vi "RH_PPMU_SetVoltage.vi"(8 "error in":errorcluster, 9 "voltage level (V)":dbl, 10 "channel list":string, 11 "PPMU Session In":refnum<k15>) -> (0 "error out":errorcluster, 3 "PPMU Session Out":refnum<k15>)   [LabVIEW 2023, in "ResourceHandling.lvlib"]
doc: "Set Voltage level"
uses:
  ResourceHandling.lvlib
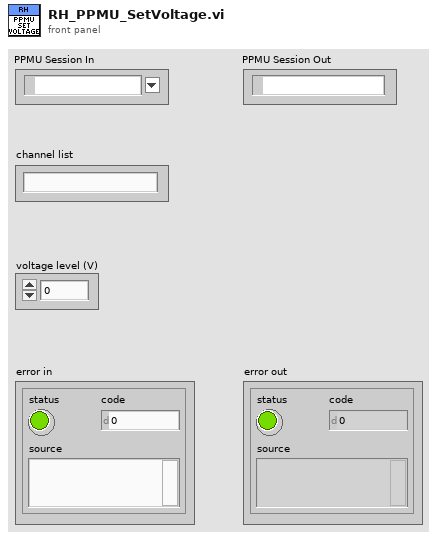
[diagram p1: front panel]
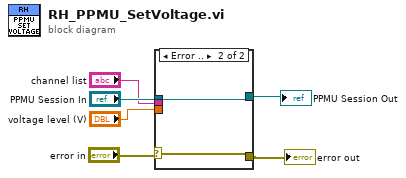
[diagram p0: block diagram]
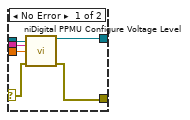
[diagram p2: hidden frame]
diagram:
  n1 = case shown="Error .." "error in" {
    selector: "error in" -> [w9 w13]
    tunnel: "PPMU Session In" -> [w12 w14]
    tunnel: "channel list" -> [w11 _]
    tunnel: "voltage level (V)" -> [w10 _]
    tunnel: [w8 w13] -> w2
    tunnel: [w7 w14] -> w1
    frame No Error {
      n2 = call <instrlib>:"niDigital PPMU Configure Voltage Level.vi"("instrument handle"=w12, "channel list"=w11, "voltage level (V)"=w10, "error in"=w9) -> ("instrument handle out"=w7:refnum<k15>, "error out"=w8:errorcluster)  [unwired: 10 in]
    }
    frame Error {
    }
  }
  "PPMU Session Out" <- w1
  "error out" <- w2
